vi "外部IO中断实验.vi"   [LabVIEW 2011]
uses:
  <vilib>/STM32_DriverVI_Interface_F4/GPIO/pin_in_F4.ctl
  <vilib>/STM32_DriverVI_Interface_F4/Interrupt/IO Interrupt Channel_F4.ctl
  <vilib>/STM32_DriverVI_Interface_F4/Interrupt/PreemptionPriority_2_F4.ctl
  <vilib>/STM32_DriverVI_Interface_F4/GPIO/PortX_in_F4.ctl
  <vilib>/STM32_DriverVI_Interface_F4/GPIO/GPI_Mode_Interface_F4.ctl
  <vilib>/STM32_DriverVI_Interface_F4/Interrupt/IO Trigger type_F4.ctl
  <vilib>/STM32_DriverVI_Interface_F4/Interrupt/SubPriority_2_F4.ctl
  <vilib>/STM32_DriverVI_Interface_F4/Interrupt/IO Priority Set_2_F4.vi
types:
  T1 = typedef "中断使能禁止_F4.ctl" = enum8{"Disable", "Enable"}
  T2 = typedef "SubPriority_2_F4.ctl" = enum8{"Priority_0（High）", "Priority_1", "Priority_2", "Priority_3（Low）"}
  T3 = typedef "PreemptionPriority_2_F4.ctl" = enum8{"Priority_0（Highest）", "Priority_1", "Priority_2", "Priority_3（Lowest）"}
  T4 = typedef "IO Interrupt Channel_F4.ctl" = u8
  T5 = typedef "IO Trigger type_F4.ctl" = enum8{"Any level Trigger", "Falling edge Trigger", "Rising edge Trigger"}
  T6 = typedef "GPI_Mode_Interface_F4.ctl" = enum8{"Floating Input", "Pull-up Input", "Pull-down Input"}
  T7 = typedef "pin_in_F4.ctl" = enum8{"P0", "P1", "P2", "P3", "P4", "P5", "P6", "P7", "P8", "P9", "P10", "P11", "P12", "P13", "P14", "P15"}
  T8 = typedef "PortX_in_F4.ctl" = enum8{"Port_A", "Port_B", "Port_C", "Port_D", "Port_E", "Port_F", "Port_G", "Port_H", "Port_I"}
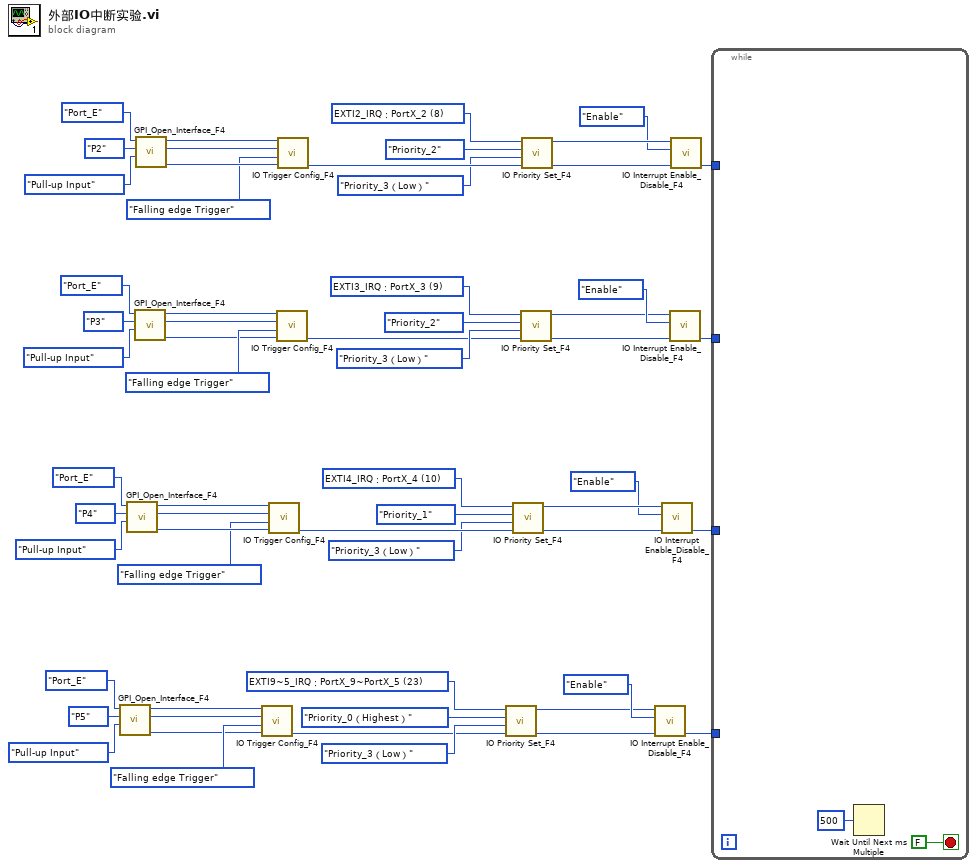
[diagram p0: block diagram]
diagram:
  w13 = T4 23 items=["EXTI0_IRQ：PortX_0"=6, "EXTI1_IRQ：PortX_1"=7, "EXTI2_IRQ：PortX_2"=8, "EXTI3_IRQ：PortX_3"=9, "EXTI4_IRQ：PortX_4"=10, "EXTI9~5_IRQ：PortX_9~PortX_5"=23, "EXTI15~10_IRQ：PortX_15~PortX_10"=40] ("IO 中断号选择")
  w24 = T4 10 items=["EXTI0_IRQ：PortX_0"=6, "EXTI1_IRQ：PortX_1"=7, "EXTI2_IRQ：PortX_2"=8, "EXTI3_IRQ：PortX_3"=9, "EXTI4_IRQ：PortX_4"=10, "EXTI9~5_IRQ：PortX_9~PortX_5"=23, "EXTI15~10_IRQ：PortX_15~PortX_10"=40] ("IO 中断号选择")
  w41 = T4 9 items=["EXTI0_IRQ：PortX_0"=6, "EXTI1_IRQ：PortX_1"=7, "EXTI2_IRQ：PortX_2"=8, "EXTI3_IRQ：PortX_3"=9, "EXTI4_IRQ：PortX_4"=10, "EXTI9~5_IRQ：PortX_9~PortX_5"=23, "EXTI15~10_IRQ：PortX_15~PortX_10"=40] ("IO 中断号选择")
  w52 = T4 8 items=["EXTI0_IRQ：PortX_0"=6, "EXTI1_IRQ：PortX_1"=7, "EXTI2_IRQ：PortX_2"=8, "EXTI3_IRQ：PortX_3"=9, "EXTI4_IRQ：PortX_4"=10, "EXTI9~5_IRQ：PortX_9~PortX_5"=23, "EXTI15~10_IRQ：PortX_15~PortX_10"=40] ("IO 中断号选择")
  n1 = call <vilib>:"GPI_Open_Interface_F4.vi"("mode"=GPI_Mode_Interface_F4."Pull-up Input", "pin_in"=pin_in_F4."P5", "PortX_in"=PortX_in_F4."Port_E") -> ("err out"=w10:u8, "pin_out"=w9:u16, "PortX_out"=w8:u16)  [unwired: 6 in]
  n2 = call <vilib>:"GPI_Open_Interface_F4.vi"("mode"=GPI_Mode_Interface_F4."Pull-up Input", "pin_in"=pin_in_F4."P4", "PortX_in"=PortX_in_F4."Port_E") -> ("err out"=w27:u8, "pin_out"=w28:u16, "PortX_out"=w29:u16)  [unwired: 6 in]
  n3 = call <vilib>:"GPI_Open_Interface_F4.vi"("mode"=GPI_Mode_Interface_F4."Pull-up Input", "pin_in"=pin_in_F4."P3", "PortX_in"=PortX_in_F4."Port_E") -> ("err out"=w38:u8, "pin_out"=w37:u16, "PortX_out"=w36:u16)  [unwired: 6 in]
  n4 = call <vilib>:"GPI_Open_Interface_F4.vi"("mode"=GPI_Mode_Interface_F4."Pull-up Input", "pin_in"=pin_in_F4."P2", "PortX_in"=PortX_in_F4."Port_E") -> ("err out"=w55:u8, "pin_out"=w56:u16, "PortX_out"=w57:u16)  [unwired: 6 in]
  n5 = call <vilib>:"IO Trigger Config_F4.vi"("err_in"=w10, "Trigger type"=IO_Trigger_type_F4."Falling edge Trigger", "pin_in"=w9, "PortX_in"=w8) -> ("err_out"=w12:u8)  [unwired: 7 in]
  n6 = call <vilib>:"IO Trigger Config_F4.vi"("err_in"=w27, "Trigger type"=IO_Trigger_type_F4."Falling edge Trigger", "pin_in"=w28, "PortX_in"=w29) -> ("err_out"=w25:u8)  [unwired: 7 in]
  n7 = call <vilib>:"IO Trigger Config_F4.vi"("err_in"=w38, "Trigger type"=IO_Trigger_type_F4."Falling edge Trigger", "pin_in"=w37, "PortX_in"=w36) -> ("err_out"=w40:u8)  [unwired: 7 in]
  n8 = call <vilib>:"IO Trigger Config_F4.vi"("err_in"=w55, "Trigger type"=IO_Trigger_type_F4."Falling edge Trigger", "pin_in"=w56, "PortX_in"=w57) -> ("err_out"=w53:u8)  [unwired: 7 in]
  n9 = call-poly <vilib>:"IO Priority Set_F4.vi"("err_in"=w12, "响应优先级"=SubPriority_2_F4."Priority_3（Low）", "抢占优先级"=PreemptionPriority_2_F4."Priority_0（Highest）", "IO 中断号设置"=w13) -> ("err_out"=w16:u8, "中断号"=w17:u16)  [unwired: 6 in]
  n10 = call-poly <vilib>:"IO Priority Set_F4.vi"("err_in"=w25, "响应优先级"=SubPriority_2_F4."Priority_3（Low）", "抢占优先级"=PreemptionPriority_2_F4."Priority_1", "IO 中断号设置"=w24) -> ("err_out"=w21:u8, "中断号"=w20:u16)  [unwired: 6 in]
  n11 = call-poly <vilib>:"IO Priority Set_F4.vi"("err_in"=w40, "响应优先级"=SubPriority_2_F4."Priority_3（Low）", "抢占优先级"=PreemptionPriority_2_F4."Priority_2", "IO 中断号设置"=w41) -> ("err_out"=w44:u8, "中断号"=w45:u16)  [unwired: 6 in]
  n12 = call-poly <vilib>:"IO Priority Set_F4.vi"("err_in"=w53, "响应优先级"=SubPriority_2_F4."Priority_3（Low）", "抢占优先级"=PreemptionPriority_2_F4."Priority_2", "IO 中断号设置"=w52) -> ("err_out"=w49:u8, "中断号"=w48:u16)  [unwired: 6 in]
  n13 = call <vilib>:"IO Interrupt Enable_Disable_F4.vi"("err_in"=w16, "中断使能禁止"=中断使能禁止_F4."Enable", "中断号"=w17) -> ("err_out"=w1:u8)  [unwired: 8 in]
  n14 = call <vilib>:"IO Interrupt Enable_Disable_F4.vi"("err_in"=w21, "中断使能禁止"=中断使能禁止_F4."Enable", "中断号"=w20) -> ("err_out"=w2:u8)  [unwired: 8 in]
  n15 = call <vilib>:"IO Interrupt Enable_Disable_F4.vi"("err_in"=w44, "中断使能禁止"=中断使能禁止_F4."Enable", "中断号"=w45) -> ("err_out"=w3:u8)  [unwired: 8 in]
  n16 = call <vilib>:"IO Interrupt Enable_Disable_F4.vi"("err_in"=w49, "中断使能禁止"=中断使能禁止_F4."Enable", "中断号"=w48) -> ("err_out"=w4:u8)  [unwired: 8 in]
  n17 = while {
    tunnel: w4 -> [_]
    tunnel: w3 -> [_]
    tunnel: w2 -> [_]
    tunnel: w1 -> [_]
    stop <- FALSE stop-if-true
    n18 = Wait Until Next ms Multiple(millisecond multiple=u32 500 ("毫秒倍数")) -> ()  [unwired: 1 out]
  }
